vi "Main.vi"() -> ()   [LabVIEW 2013]
uses:
  <vilib>/myRIO/Instrument Drivers/Onboard IO/I2C/typedefs/I2C User Configuration.ctl
  <vilib>/myRIO/Instrument Drivers/Onboard IO/I2C/typedefs/I2C Transfer Rate.ctl
  <vilib>/Platform/TimedLoop/XDataNode/timing_clust.ctl
  <vilib>/Platform/TimedLoop/XDataNode/nitl_modes.ctl
  <vilib>/Platform/TimedLoop/XDataNode/wakeup.ctl
  <vilib>/myRIO/Common/Instrument Driver Framework/myRIO v1.0/I2C/vis/myRIO v1.1 Open I2C.vi
  <vilib>/myRIO/Common/Instrument Driver Framework/myRIO v1.0/UART/vis/myRIO v1.0 Close UART.vi
  <vilib>/myRIO/Common/Instrument Driver Framework/Utilities/vis/Validate Channels.vi
  <vilib>/myRIO/Common/Instrument Driver Framework/myRIO v1.0/I2C/vis/myRIO v1.0 Reserve I2C.vi
  <vilib>/myRIO/Common/Instrument Driver Framework/myRIO v1.0/I2C/vis/myRIO v1.0 Build MUX Configuration I2C.vi
  <vilib>/myRIO/Common/Instrument Driver Framework/myRIO v1.0/Resource Manager/vis/myRIO v1.0 Reserve Channel List.vi
  <vilib>/myRIO/Common/Instrument Driver Framework/myRIO v1.0/Resource Manager/vis/myRIO v1.0 Create Configuration List.vi
  <vilib>/myRIO/Common/Instrument Driver Framework/myRIO v1.0/Resource Manager/vis/myRIO v1.0 Reserve Channel.vi
  <vilib>/myRIO/Common/Instrument Driver Framework/myRIO v1.0/Resource Manager/vis/myRIO v1.0 Unreserve Channel.vi
  <vilib>/myRIO/Common/Instrument Driver Framework/myRIO v1.0/Resource Manager/vis/myRIO v1.0 Build Mutex Name.vi
  <vilib>/myRIO/Common/Instrument Driver Framework/myRIO v1.0/myRIO v1.1 Open.vi
  <vilib>/Utility/VariantDataType/GetNumericInfo.vi
  <vilib>/Utility/error.llb/Error Cluster From Error Code.vi
  <vilib>/myRIO/Common/Instrument Driver Framework/Utilities/vis/IO Manager.vi
  <vilib>/myRIO/Common/Instrument Driver Framework/Utilities/vis/Configuration Manager.vi
  <vilib>/myRIO/Common/Instrument Driver Framework/myRIO v1.0/Resource Manager/vis/myRIO v1.0 Configure IO.vi
  <vilib>/myRIO/Common/Instrument Driver Framework/myRIO v1.0/myRIO v1.0 Close.vi
  <vilib>/myRIO/Common/Instrument Driver Framework/myRIO v1.0/I2C/vis/myRIO v1.0 Configure I2C.vi
  <vilib>/myRIO/Common/Instrument Driver Framework/myRIO v1.0/I2C/vis/myRIO v1.0 Write I2C.vi
  <vilib>/myRIO/Common/Instrument Driver Framework/myRIO v1.0/I2C/vis/myRIO v1.0 Read I2C.vi
  <vilib>/myRIO/Common/Instrument Driver Framework/Utilities/vis/FPGA Ref Manager.vi
  <vilib>/myRIO/Common/Instrument Driver Framework/myRIO v1.0/myRIO v1.0 Reset FPGA.vi
  <vilib>/platform/TimedLoop/XDataNode/XDataNode.xnode
  <vilib>/myRIO/Instrument Drivers/Utilities/Utilities.lvlib
  <vilib>/myRIO/Instrument Drivers/Onboard IO/I2C/I2C.lvlib
  <vilib>/Platform/TimedLoop/XDataNode/XDNodeRunTimeDep.lvlib
panel:
  out "X":i16
  out "Y":i16
  out "Z":i16
  out "Accelerometer: Waveform Chart 3":cluster{i16, i16, i16}(graph)
  out "X rate":i16
  out "Y rate":i16
  out "Z rate":i16
  out "Gyroscope: Angular rate [LSB/sec] 2":cluster{i16, i16, i16}(graph)
  out "X 3":i16
  out "Y 3":i16
  out "Z 3":i16
  out "Compass: Magnetic field [LSb]  2":cluster{i16, i16, i16}(graph) caption="Waveform Chart"
  out "Accelerometer: Waveform Chart":cluster{i16, i16, i16}(graph)
  out "Z":i16
  out "Y":i16
  out "X":i16
  in  "[ESC]":bool
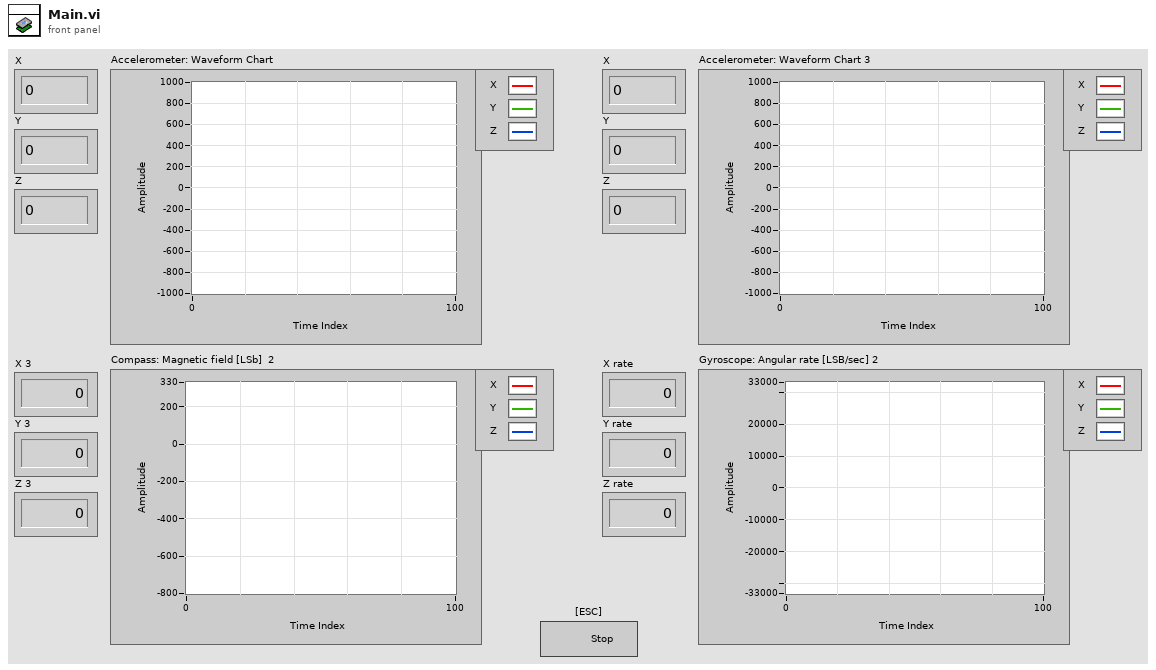
[diagram p1: front panel]
types:
  T1 = typedef "I2C.lvlib/I2C User Configuration.ctl" = cluster{"I2C Transfer Rate":T2}
  T2 = typedef "I2C.lvlib/I2C Transfer Rate.ctl" = enum16{"Standard Mode (100 kbps)", "Fast Mode (400 kbps)"}
  T3 = typedef "I2C.lvlib/I2C Reference.ctl" = cluster{"myRIO Reference":T4, "I2C Channels Enum":T8, "I2C Configuration":T9}
  T4 = typedef "myRIO Generic Hardware Reference.ctl" = cluster{"myRIO Model":T5, "myRIO Hardware Reference":T6}
  T5 = typedef "Hardware Version Enum.ctl" = enum16{"Unknown", "myRIO-1900", "myRIO-1950"}
  T6 = typedef "myRIO v1.0 Reference.ctl" = cluster{"Generic FPGA Reference":T7, "Allow multiple opens":bool}
  T7 = typedef "Generic FPGA Reference.ctl" = refnum<k20>
  T8 = typedef "I2C Channels Enum.ctl" = enum16{"Not Connected", "A/I2C", "B/I2C"}
  T9 = typedef "I2C.lvlib/I2C Configuration.ctl" = cluster{"I2C Transfer Rate":T2}
  T10 = typedef "XDNodeRunTimeDep.lvlib/timing_clust.ctl" = cluster{"Expected End [f-1]":u64, "Actual End [f-1]":u64, "Finished Late? [f-1]":bool, "Expected End [i-1]":u64, "Actual End [i-1]":u64, "Finished Late? [i-1]":bool, "Expected Start [i]":u64, "Actual Start [i]":u64, "Expected Start [f]":u64, "Actual Start [f]":u64, "Source Name":string, "Structure Name":string, "Period":i64, "Deadline":i64, "Offset":i64, "Start":i64, "Priority":i32, "Timeout":i32, "Mode":T11, "Wakeup Reason":T12, "Error":errorcluster, "Source Type":string, "Secondary Source Type":string, "Global End Time":u64, "Global Start Time":u64, "Frame Duration":u64, "Iteration Duration":u64, "Assigned CPU":i32, "I/O Scan Engine Mode":u32}
  T11 = typedef "XDNodeRunTimeDep.lvlib/nitl_modes.ctl" = enum32{"No Change", "Process missed periods, maintain original phase", "Discard missed periods, maintain original phase", "Process missed periods, ignore original phase", "Discard missed periods, ignore original phase"}
  T12 = typedef "XDNodeRunTimeDep.lvlib/wakeup.ctl" = enum32{"Normal", "Aborted", "Asynchronous wakeup", "Timing source error", "Timed loop error", "Timeout"}
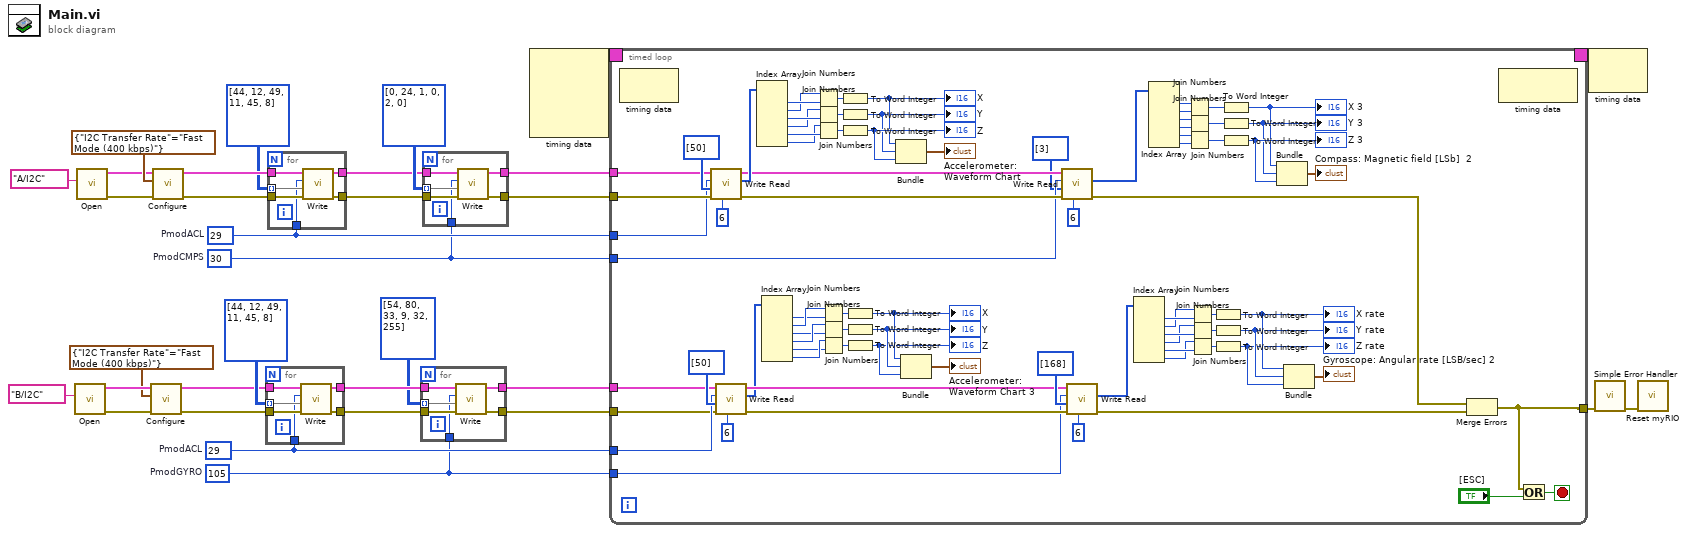
[diagram p0: block diagram]
diagram:
  w3 = u8 105  # PmodGYRO
  w4 = u8 29  # PmodACL
  w16 = u8 30  # PmodCMPS
  w17 = u8 29  # PmodACL
  n1 = call <vilib>:"Open.vi"("Channel Name"=tag "B/I2C" ("I2C channel")) -> ("error out"=w10:errorcluster, "I2C Ref Out"=w9:T3)  [unwired: 9 in]
  n2 = call <vilib>:"Open.vi"("Channel Name"=tag "A/I2C" ("I2C channel")) -> ("error out"=w28:errorcluster, "I2C Ref Out"=w29:T3)  [unwired: 9 in]
  n3 = call <vilib>:"Configure.vi"("error in (no error)"=w10, "I2C User Configuration"=T1 {"I2C Transfer Rate"=enum."Fast Mode (400 kbps)"} ("I2C bus speed"), "I2C Ref In"=w9) -> ("error out"=w12:errorcluster, "I2C Ref Out"=w11:T3)  [unwired: 7 in]
  n4 = call <vilib>:"Configure.vi"("error in (no error)"=w28, "I2C User Configuration"=T1 {"I2C Transfer Rate"=enum."Fast Mode (400 kbps)"} ("I2C bus speed"), "I2C Ref In"=w29) -> ("error out"=w26:errorcluster, "I2C Ref Out"=w27:T3)  [unwired: 7 in]
  n5 = for {
    tunnel: [w38] -> w15
    tunnel: [w37] -> w14
    tunnel: u8[][] [[44, 12], [49, 11], [45, 8]] ("Bytes to Write") -> [w36] mode=indexing
    tunnel: w11 -> [w35]
    tunnel: w12 -> [w34]
    tunnel: w4 -> [w33]
    n6 = call <vilib>:"Write.vi"("error in (no error)"=w34, "Bytes to Write"=w36, "Slave Address (7-bit)"=w33, "I2C Ref In"=w35) -> ("error out"=w38:errorcluster, "I2C Ref Out"=w37:T3)  [unwired: 6 in]
  }
  n7 = for {
    tunnel: [w44] -> w18
    tunnel: [w43] -> w19
    tunnel: u8[][] [[44, 12], [49, 11], [45, 8]] ("Bytes to Write") -> [w42] mode=indexing
    tunnel: w27 -> [w41]
    tunnel: w26 -> [w40]
    tunnel: w17 -> [w39]
    n8 = call <vilib>:"Write.vi"("error in (no error)"=w40, "Bytes to Write"=w42, "Slave Address (7-bit)"=w39, "I2C Ref In"=w41) -> ("error out"=w44:errorcluster, "I2C Ref Out"=w43:T3)  [unwired: 6 in]
  }
  n9 = for {
    tunnel: [w50] -> w5
    tunnel: [w49] -> w6
    tunnel: u8[][] [[54, 80], [33, 9], [32, 255]] ("Bytes to Write") -> [w48] mode=indexing
    tunnel: w14 -> [w47]
    tunnel: w15 -> [w46]
    tunnel: w3 -> [w45]
    n10 = call <vilib>:"Write.vi"("error in (no error)"=w46, "Bytes to Write"=w48, "Slave Address (7-bit)"=w45, "I2C Ref In"=w47) -> ("error out"=w50:errorcluster, "I2C Ref Out"=w49:T3)  [unwired: 6 in]
  }
  n11 = for {
    tunnel: [w56] -> w20
    tunnel: [w55] -> w21
    tunnel: u8[][] [[0, 24], [1, 0], [2, 0]] ("Bytes to Write") -> [w54] mode=indexing
    tunnel: w19 -> [w53]
    tunnel: w18 -> [w52]
    tunnel: w16 -> [w51]
    n12 = call <vilib>:"Write.vi"("error in (no error)"=w52, "Bytes to Write"=w54, "Slave Address (7-bit)"=w51, "I2C Ref In"=w53) -> ("error out"=w56:errorcluster, "I2C Ref Out"=w55:T3)  [unwired: 6 in]
  }
  n13 = node-c288() -> (w25:T10)  [unwired: 4 in]
  n14 = timed-loop {
    tunnel: w20 -> [w118]
    tunnel: w21 -> [w119]
    timing: w25 -> [_]
    timing-out: [_] -> w24
    tunnel: w17 -> [w117]
    tunnel: w16 -> [w99]
    tunnel: w6 -> [w60]
    tunnel: w5 -> [w61]
    tunnel: w4 -> [w62]
    tunnel: w3 -> [w63]
    tunnel: [w58] -> w2
    stop <- w137 stop-if-true
    n15 = node-c288() -> ()  [unwired: 1 in, 1 out]
    n16 = call <vilib>:"Write Read.vi"("Byte Count"=u32 6, "error in (no error)"=w118, "Bytes to Write"=u8[] [50], "Slave Address (7-bit)"=w117, "I2C Ref In"=w119) -> ("error out"=w100:errorcluster, "Bytes Read"=w120:u8[], "I2C Ref Out"=w101:T3)  [unwired: 3 in]
    n17 = call <vilib>:"Write Read.vi"("Byte Count"=u32 6, "error in (no error)"=w61, "Bytes to Write"=u8[] [50], "Slave Address (7-bit)"=w62, "I2C Ref In"=w60) -> ("error out"=w82:errorcluster, "Bytes Read"=w79:u8[], "I2C Ref Out"=w81:T3)  [unwired: 3 in]
    n18 = Index Array(array=w120) -> (element #1=w128:u8, element #2=w127:u8, element #3=w126:u8, element #4=w125:u8, element #5=w124:u8, element #6=w123:u8)  [unwired: 6 in]
    n19 = Index Array(array=w79) -> (element #1=w71:u8, element #2=w72:u8, element #3=w73:u8, element #4=w74:u8, element #5=w75:u8, element #6=w76:u8)  [unwired: 6 in]
    n20 = Join Numbers(hi=w127, lo=w128) -> ((hi.lo)=w135:u16)
    n21 = Join Numbers(hi=w125, lo=w126) -> ((hi.lo)=w134:u16)
    n22 = Join Numbers(hi=w123, lo=w124) -> ((hi.lo)=w133:u16)
    n23 = Join Numbers(hi=w72, lo=w71) -> ((hi.lo)=w64:u16)
    n24 = Join Numbers(hi=w74, lo=w73) -> ((hi.lo)=w65:u16)
    n25 = Join Numbers(hi=w76, lo=w75) -> ((hi.lo)=w66:u16)
    n26 = To Word Integer(number=w135) -> (16bit integer=w130:i16)
    "X" <- w130
    n27 = To Word Integer(number=w134) -> (16bit integer=w129:i16)
    "Y" <- w129
    n28 = To Word Integer(number=w133) -> (16bit integer=w132:i16)
    "Z" <- w132
    n29 = To Word Integer(number=w64) -> (16bit integer=w69:i16)
    "X" <- w69
    n30 = To Word Integer(number=w65) -> (16bit integer=w70:i16)
    "Y" <- w70
    n31 = To Word Integer(number=w66) -> (16bit integer=w67:i16)
    "Z" <- w67
    n32 = Bundle(w130, w129, w132) -> (→"Accelerometer: Waveform Chart":cluster{i16, i16, i16})  [unwired: 1 in]
    n33 = Bundle(w69, w70, w67) -> (→"Accelerometer: Waveform Chart 3":cluster{i16, i16, i16})  [unwired: 1 in]
    n34 = call <vilib>:"Write Read.vi"("Byte Count"=u32 6, "error in (no error)"=w100, "Bytes to Write"=u8[] [3], "Slave Address (7-bit)"=w99, "I2C Ref In"=w101) -> ("error out"=w57:errorcluster, "Bytes Read"=w106:u8[])  [unwired: 3 in, 1 out]
    n35 = call <vilib>:"Write Read.vi"("Byte Count"=u32 6, "error in (no error)"=w82, "Bytes to Write"=u8[] [168], "Slave Address (7-bit)"=w63, "I2C Ref In"=w81) -> ("error out"=w59:errorcluster, "Bytes Read"=w97:u8[])  [unwired: 3 in, 1 out]
    n36 = Index Array(array=w97) -> (element #1=w92:u8, element #2=w91:u8, element #3=w90:u8, element #4=w89:u8, element #5=w88:u8, element #6=w87:u8)  [unwired: 6 in]
    n37 = Index Array(array=w106) -> (element #1=w111:u8, element #2=w112:u8, element #3=w113:u8, element #4=w114:u8, element #5=w115:u8, element #6=w116:u8)  [unwired: 6 in]
    n38 = Join Numbers(hi=w111, lo=w112) -> ((hi.lo)=w102:u16)
    n39 = Join Numbers(hi=w113, lo=w114) -> ((hi.lo)=w103:u16)
    n40 = Join Numbers(hi=w115, lo=w116) -> ((hi.lo)=w104:u16)
    n41 = Join Numbers(hi=w91, lo=w92) -> ((hi.lo)=w96:u16)
    n42 = Join Numbers(hi=w89, lo=w90) -> ((hi.lo)=w95:u16)
    n43 = Join Numbers(hi=w87, lo=w88) -> ((hi.lo)=w94:u16)
    n44 = To Word Integer(number=w96) -> (16bit integer=w86:i16)
    "X rate" <- w86
    n45 = To Word Integer(number=w95) -> (16bit integer=w85:i16)
    "Y rate" <- w85
    n46 = To Word Integer(number=w94) -> (16bit integer=w84:i16)
    "Z rate" <- w84
    n47 = To Word Integer(number=w102) -> (16bit integer=w107:i16)
    "X 3" <- w107
    n48 = To Word Integer(number=w103) -> (16bit integer=w108:i16)
    "Y 3" <- w108
    n49 = To Word Integer(number=w104) -> (16bit integer=w109:i16)
    "Z 3" <- w109
    n50 = Bundle(w107, w108, w109) -> (→"Compass: Magnetic field [LSb]  2":cluster{i16, i16, i16})  [unwired: 1 in]
    n51 = Bundle(w86, w85, w84) -> (→"Gyroscope: Angular rate [LSB/sec] 2":cluster{i16, i16, i16})  [unwired: 1 in]
    n52 = Merge Errors(w57, w59) -> (w58:errorcluster)
    n53 = node-c288() -> ()  [unwired: 1 in, 1 out]
    n54 = Or(x=w58, y="[ESC]") -> (x .or. y?=w137:bool)
  }
  n55 = node-c288(w24) -> ()  [unwired: 1 out]
  n56 = call <vilib>:"Simple Error Handler.vi"("error in (no error)"=w2) -> ("error out"=w32:errorcluster)  [unwired: 4 in, 4 out]
  n57 = call <vilib>:"Reset myRIO.vi"("error in (no error)"=w32) -> ()  [unwired: 10 in, 1 out]
